vi "BuildUI.vi"(8 "error in (no error)":errorcluster, 11 "reference in":refnum<class "AbstractBuilder.lvclass">) -> (0 "error out":errorcluster, 3 "reference out":refnum<class "AbstractBuilder.lvclass">)   [LabVIEW 2015, in "AbstractBuilder.lvclass"]
uses:
  AbstractBuilder.lvclass
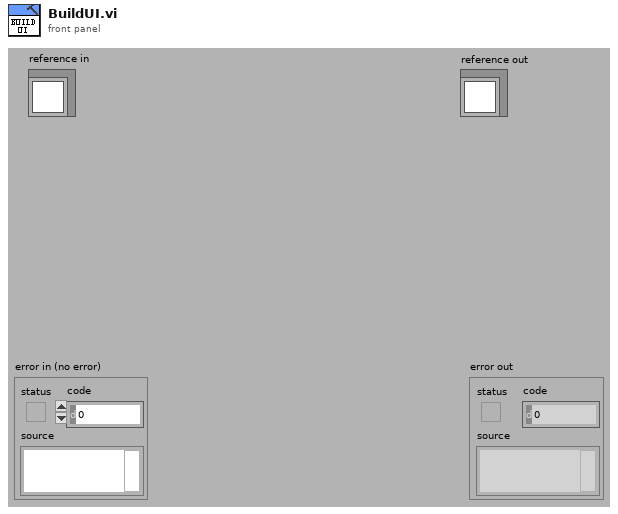
[diagram p1: front panel]
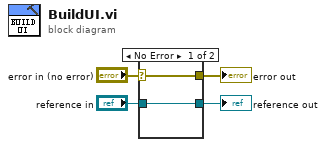
[diagram p0: block diagram]
diagram:
  n1 = case shown="No Error" "error in (no error)" {
    selector: "error in (no error)" -> [w5 w8]
    tunnel: [w5 w8] -> w3
    tunnel: [w6 w7] -> w1
    tunnel: "reference in" -> [w6 w7]
    frame No Error {
    }
    frame Error {
    }
  }
  "error out" <- w3
  "reference out" <- w1
